vi "FindControl.vi"(5 "Control":refnum<class "Control.lvclass">, 6 "error in":errorcluster, 9 "Page in":refnum<class "Page.lvclass">) -> (0 "error out":errorcluster, 3 "Page out":refnum<class "Page.lvclass">, 4 "On page":bool)   [LabVIEW 2014, in "Page.lvclass"]
uses:
  Page.lvclass
  Control/Control.lvclass
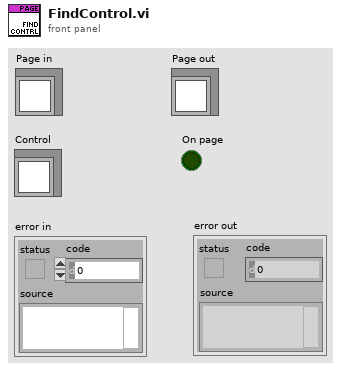
[diagram p1: front panel]
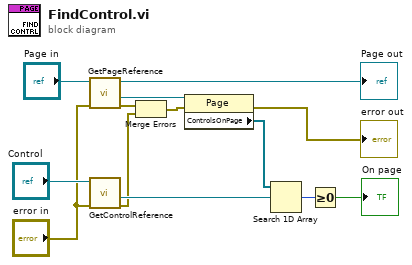
[diagram p0: block diagram]
diagram:
  n1 = call "GetPageReference.vi"("error in"="error in", "Page in"="Page in") -> ("error out"=w2:errorcluster, "page reference"=w10:refnum<vi>, "Page out"=→"Page out":refnum<class "Page.lvclass">)  [unwired: 7 in]
  n2 = call "GetControlReference.vi"("error in"="error in", "Control in"="Control") -> ("error out"=w3:errorcluster, "control reference"=w8:refnum<vi>)  [unwired: 7 in, 1 out]
  n3 = Merge Errors(w2, w3) -> (w1:errorcluster)
  n4 = property class="Page"(reference=w10, error in=w1) -> (error out=→"error out":errorcluster, "ControlsOnPage"=w9:refnum<vi>[])  [unwired: 1 out]
  n5 = Search 1D Array(1D array=w9, element=w8) -> (index of element=w6:i32)  [unwired: 1 in]
  n6 = Greater Or Equal To 0?(x=w6) -> (x >= 0?=→"On page":bool)
